vi "Stop Core.vi"(10 "final error code":i32, 11 "Camera_Controller in":refnum<class "Camera_Controller.lvclass">) -> (3 "Camera_Controller out":refnum<class "Camera_Controller.lvclass">)   [LabVIEW 2023, in "Camera_Controller.lvlib" / "Camera_Controller.lvclass"]
doc: "(<B>Filename</B>: Actor Framework.lvlib:Actor.lvclass:Stop Core.vi)\n\nDefines what the actor does before it stops. Use the <B>final error code</B> input to determine whether the actor shut down in response to an error.\n\nBy default, this method passes the Stop message along to all auto-stop nested actors. A descendant class may override this method to define additional behavior, such as shutting down any processes the actor initiated in its override of the Actor Core method."
uses:
  Camera_Controller.lvclass
  Camera_Controller.lvclass/Camera_Controller.ctl
  <vilib>/ActorFramework/Actor/Actor.lvclass
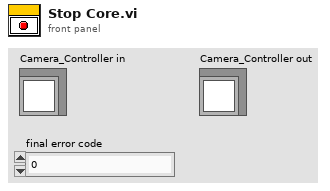
[diagram p1: front panel]
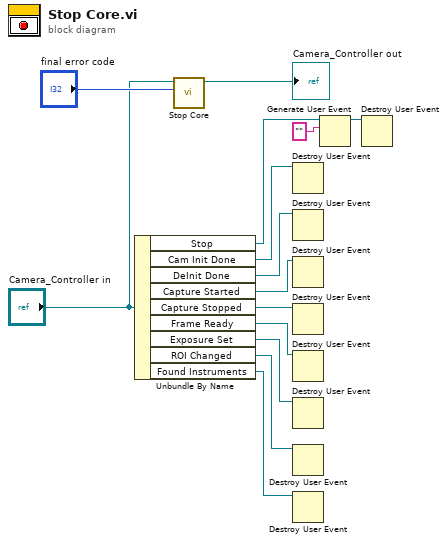
[diagram p0: block diagram]
diagram:
  n1 = Unbundle By Name("Camera_Controller in") -> ("Stop"=w12:refnum<user-event>, "Cam Init Done"=w8:refnum<user-event>, "DeInit Done"=w7:refnum<user-event>, "Capture Started"=w4:refnum<user-event>, "Capture Stopped"=w5:refnum<user-event>, "Frame Ready"=w3:refnum<user-event>, "Exposure Set"=w6:refnum<user-event>, "ROI Changed"=w2:refnum<user-event>, "Found Instruments"=w1:refnum<user-event>)
  n2 = call-parent "Stop Core.vi"("final error code"="final error code", "Actor in"="Camera_Controller in") -> ("Actor out"=→"Camera_Controller out":refnum<class "Camera_Controller.lvclass">)  [unwired: 9 in]
  n3 = Destroy User Event(user event=w8) -> ()  [unwired: 1 in, 1 out]
  n4 = Destroy User Event(user event=w7) -> ()  [unwired: 1 in, 1 out]
  n5 = Destroy User Event(user event=w4) -> ()  [unwired: 1 in, 1 out]
  n6 = Destroy User Event(user event=w5) -> ()  [unwired: 1 in, 1 out]
  n7 = Destroy User Event(user event=w3) -> ()  [unwired: 1 in, 1 out]
  n8 = Destroy User Event(user event=w6) -> ()  [unwired: 1 in, 1 out]
  n9 = Destroy User Event(user event=w2) -> ()  [unwired: 1 in, 1 out]
  n10 = Destroy User Event(user event=w1) -> ()  [unwired: 1 in, 1 out]
  n11 = Generate User Event(user event=w12, event data cluster="" ("event data")) -> (user event out=w9:refnum<user-event>)  [unwired: 2 in, 1 out]
  n12 = Destroy User Event(user event=w9) -> ()  [unwired: 1 in, 1 out]
